vi "AudioTest.Calibrate Generated Waveform, Scale Amplitude based on Frequency.vi"(8 "error in (no error)":errorcluster, 10 "Calibration File":path=path "C:/MTE/Utah Core Audio Test/Config/Speaker Calibration, PN XXX, SN YYY, v10-30-18.csv", 11 "Frequencies and Amplitudes":T1(array[cluster])=[{"frequency [Hz]"=100.0, "amplitude [V]"=1.0}, {"frequency [Hz]"=104.55297296988265, "amplitude [V]"=1.0}, {"frequency [Hz]"=109.31324156841022, "amplitude [V]"=1.0}, {"frequency [Hz]"=114.29024390952246, "amplitude [V]"=1.0}, {"frequency [Hz]"=119.49384782193596, "amplitude [V]"=1.0}, {"frequency [Hz]"=124.93437041394141, "amplitude [V]"=1.0}, {"frequency [Hz]"=130.62259852898134, "amplitude [V]"=1.0}, {"frequency [Hz]"=136.56981013256419, "amplitude [V]"=1.0}, {"frequency [Hz]"=142.78779667291988, "amplitude [V]"=1.0}, {"frequency [Hz]"=149.28888645972907, "amplitude [V]"=1.0}, {"frequency [Hz]"=156.08596910727934, "amplitude [V]"=1.0}, {"frequency [Hz]"=163.19252109051314, "amplitude [V]"=1.0}, {"frequency [Hz]"=170.62263246463442, "amplitude [V]"=1.0}, {"frequency [Hz]"=178.39103480125144, "amplitude [V]"=1.0}, {"frequency [Hz]"=186.51313039644634, "amplitude [V]"=1.0}, {"frequency [Hz]"=195.00502280867852, "amplitude [V]"=1.0}, {"frequency [Hz]"=203.88354878707136, "amplitude [V]"=1.0}, {"frequency [Hz]"=213.1663116533842, "amplitude [V]"=1.0}, {"frequency [Hz]"=222.87171620385857, "amplitude [V]"=1.0}, {"frequency [Hz]"=233.01900520013405, "amplitude [V]"=1.0}, {"frequency [Hz]"=243.6282975215856, "amplitude [V]"=1.0}, {"frequency [Hz]"=254.72062805472865, "amplitude [V]"=1.0}, {"frequency [Hz]"=266.31798939877575, "amplitude [V]"=1.0}, {"frequency [Hz]"=278.4433754700372, "amplitude [V]"=1.0}, {"frequency [Hz]"=291.1208270916169, "amplitude [V]"=1.0}, {"frequency [Hz]"=304.37547965879696, "amplitude [V]"=1.0}, {"frequency [Hz]"=318.233612974613, "amplitude [V]"=1.0}, {"frequency [Hz]"=332.72270335442806, "amplitude [V]"=1.0}, {"frequency [Hz]"=347.871478102818, "amplitude [V]"=1.0}, {"frequency [Hz]"=363.70997247077054, "amplitude [V]"=1.0}, {"frequency [Hz]"=380.2695892061327, "amplitude [V]"=1.0}, {"frequency [Hz]"=397.5831608153717, "amplitude [V]"=1.0}, {"frequency [Hz]"=415.6850146601006, "amplitude [V]"=1.0}, {"frequency [Hz]"=434.61104101742814, "amplitude [V]"=1.0}, {"frequency [Hz]"=454.3987642390772, "amplitude [V]"=1.0}, {"frequency [Hz]"=475.08741715036314, "amplitude [V]"=1.0}, {"frequency [Hz]"=496.7180188365328, "amplitude [V]"=1.0}, {"frequency [Hz]"=519.3334559706973, "amplitude [V]"=1.0}, {"frequency [Hz]"=542.9785678446004, "amplitude [V]"=1.0}, {"frequency [Hz]"=567.700235270821, "amplitude [V]"=1.0}, {"frequency [Hz]"=593.5474735326624, "amplitude [V]"=1.0}, {"frequency [Hz]"=620.5715295660258, "amplitude [V]"=1.0}, {"frequency [Hz]"=648.8259835659542, "amplitude [V]"=1.0}, {"frequency [Hz]"=678.3668552192873, "amplitude [V]"=1.0}, {"frequency [Hz]"=709.2527147740651, "amplitude [V]"=1.0}, {"frequency [Hz]"=741.5447991658872, "amplitude [V]"=1.0}, {"frequency [Hz]"=775.3071334314806, "amplitude [V]"=1.0}, {"frequency [Hz]"=810.6066576501887, "amplitude [V]"=1.0}, {"frequency [Hz]"=847.5133596650709, "amplitude [V]"=1.0}, {"frequency [Hz]"=886.1004138467658, "amplitude [V]"=1.0}, {"frequency [Hz]"=926.4443261752274, "amplitude [V]"=1.0}, {"frequency [Hz]"=968.6250859269978, "amplitude [V]"=1.0}, {"frequency [Hz]"=1012.7263242687566, "amplitude [V]"=1.0}, {"frequency [Hz]"=1058.8354800716002, "amplitude [V]"=1.0}, {"frequency [Hz]"=1107.0439732747873, "amplitude [V]"=1.0}, {"frequency [Hz]"=1157.4473861427032, "amplitude [V]"=1.0}, {"frequency [Hz]"=1210.1456527743937, "amplitude [V]"=1.0}, {"frequency [Hz]"=1265.2432572414218, "amplitude [V]"=1.0}, {"frequency [Hz]"=1322.8494407468877, "amplitude [V]"=1.0}, {"frequency [Hz]"=1383.0784182163372, "amplitude [V]"=1.0}, {"frequency [Hz]"=1446.0496047500092, "amplitude [V]"=1.0}, {"frequency [Hz]"=1511.8878523853718, "amplitude [V]"=1.0}, {"frequency [Hz]"=1580.723697639417, "amplitude [V]"=1.0}, {"frequency [Hz]"=1652.693620321469, "amplitude [V]"=1.0}, {"frequency [Hz]"=1727.9403141296805, "amplitude [V]"=1.0}, {"frequency [Hz]"=1806.612969567712, "amplitude [V]"=1.0}, {"frequency [Hz]"=1888.867569742524, "amplitude [V]"=1.0}, {"frequency [Hz]"=1974.8671996297824, "amplitude [V]"=1.0}, {"frequency [Hz]"=2064.7823694200047, "amplitude [V]"=1.0}, {"frequency [Hz]"=2158.7913525866, "amplitude [V]"=1.0}, {"frequency [Hz]"=2257.080539346032, "amplitude [V]"=1.0}, {"frequency [Hz]"=2359.8448062109383, "amplitude [V]"=1.0}, {"frequency [Hz]"=2467.2879023689043, "amplitude [V]"=1.0}, {"frequency [Hz]"=2579.6228536529447, "amplitude [V]"=1.0}, {"frequency [Hz]"=2697.0723849046813, "amplitude [V]"=1.0}, {"frequency [Hz]"=2819.8693615675606, "amplitude [V]"=1.0}, {"frequency [Hz]"=2948.257251385734, "amplitude [V]"=1.0}, {"frequency [Hz]"=3082.4906071239316, "amplitude [V]"=1.0}, {"frequency [Hz]"=3222.8355712654557, "amplitude [V]"=1.0}, {"frequency [Hz]"=3369.5704036889383, "amplitude [V]"=1.0}, {"frequency [Hz]"=3522.9860333700613, "amplitude [V]"=1.0}, {"frequency [Hz]"=3683.3866352021446, "amplitude [V]"=1.0}, {"frequency [Hz]"=3851.090233079168, "amplitude [V]"=1.0}, {"frequency [Hz]"=4026.429330437053, "amplitude [V]"=1.0}, {"frequency [Hz]"=4209.751569503279, "amplitude [V]"=1.0}, {"frequency [Hz]"=4401.4204205619735, "amplitude [V]"=1.0}, {"frequency [Hz]"=4601.81590260106, "amplitude [V]"=1.0}, {"frequency [Hz]"=4811.3353367702475, "amplitude [V]"=1.0}, {"frequency [Hz]"=5030.394134143814, "amplitude [V]"=1.0}, {"frequency [Hz]"=5259.426619349943, "amplitude [V]"=1.0}, {"frequency [Hz]"=5498.886891699759, "amplitude [V]"=1.0}, {"frequency [Hz]"=5749.249725523269, "amplitude [V]"=1.0}, {"frequency [Hz]"=6011.011511497396, "amplitude [V]"=1.0}, {"frequency [Hz]"=6284.691240832413, "amplitude [V]"=1.0}, {"frequency [Hz]"=6570.831534268094, "amplitude [V]"=1.0}, {"frequency [Hz]"=6869.9997179198535, "amplitude [V]"=1.0}, {"frequency [Hz]"=7182.788948107758, "amplitude [V]"=1.0}, {"frequency [Hz]"=7509.819387398822, "amplitude [V]"=1.0}, {"frequency [Hz]"=7851.739434194097, "amplitude [V]"=1.0}, {"frequency [Hz]"=8209.22700829857, "amplitude [V]"=1.0}, {"frequency [Hz]"=8582.99089502272, "amplitude [V]"=1.0}, {"frequency [Hz]"=8973.772150480592, "amplitude [V]"=1.0}, {"frequency [Hz]"=9382.345570870839, "amplitude [V]"=1.0}, {"frequency [Hz]"=9809.52122865357, "amplitude [V]"=1.0}, {"frequency [Hz]"=10256.146078669068, "amplitude [V]"=1.0}, {"frequency [Hz]"=10723.105637382549, "amplitude [V]"=1.0}, {"frequency [Hz]"=11211.32573858456, "amplitude [V]"=1.0}, {"frequency [Hz]"=11721.774369027788, "amplitude [V]"=1.0}, {"frequency [Hz]"=12255.46358764028, "amplitude [V]"=1.0}, {"frequency [Hz]"=12813.451532119352, "amplitude [V]"=1.0}, {"frequency [Hz]"=13396.84451688576, "amplitude [V]"=1.0}, {"frequency [Hz]"=14006.799226556774, "amplitude [V]"=1.0}, {"frequency [Hz]"=14644.525009287636, "amplitude [V]"=1.0}, {"frequency [Hz]"=15311.286274528236, "amplitude [V]"=1.0}, {"frequency [Hz]"=16008.404999948825, "amplitude [V]"=1.0}, {"frequency [Hz]"=16737.26335250587, "amplitude [V]"=1.0}, {"frequency [Hz]"=17499.306428843538, "amplitude [V]"=1.0}, {"frequency [Hz]"=18296.04512046572, "amplitude [V]"=1.0}, {"frequency [Hz]"=19129.059109358055, "amplitude [V]"=1.0}, {"frequency [Hz]"=20000.0, "amplitude [V]"=1.0}]) -> (0 "error out":errorcluster, 3 "Frequencies and Amplitudes Out":T1(array[cluster]))   [LabVIEW 2018]
uses:
  <vilib>/KATE/Files/File Utils.lvlib
panel:
  in  "Normal":bool=TRUE
  out "Cnt":i32
  out "XY Graph":cluster{dbl[], dbl[]}[](graph)
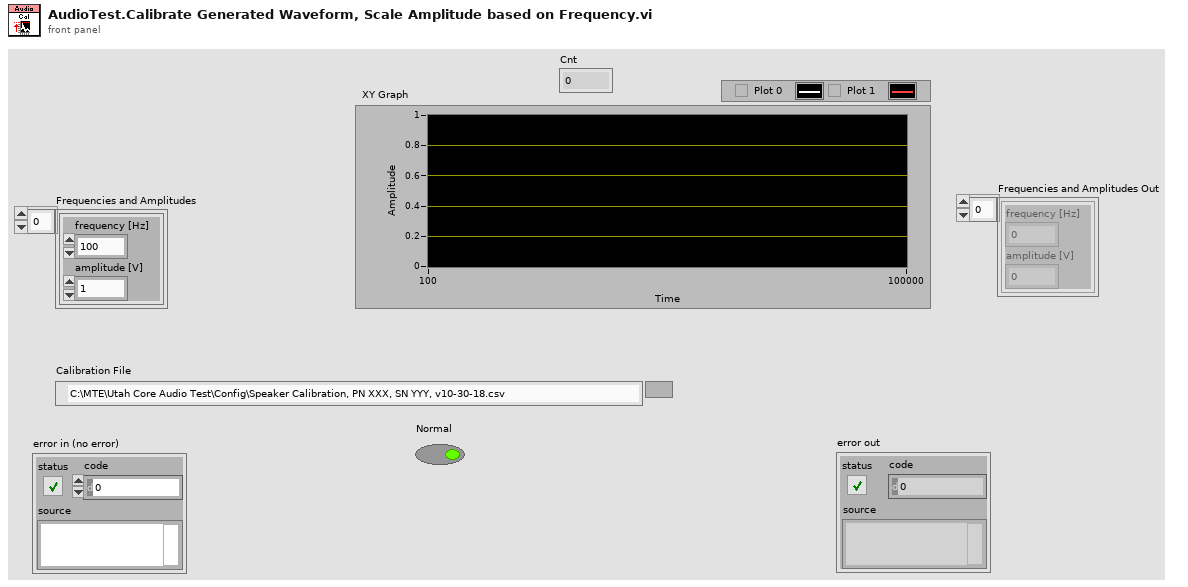
[diagram p1: front panel]
types:
  T1 = cluster{"frequency [Hz]":dbl, "amplitude [V]":dbl}[]
  T2 = cluster{"frequency [Hz]":dbl, "amplitude [V]":dbl}
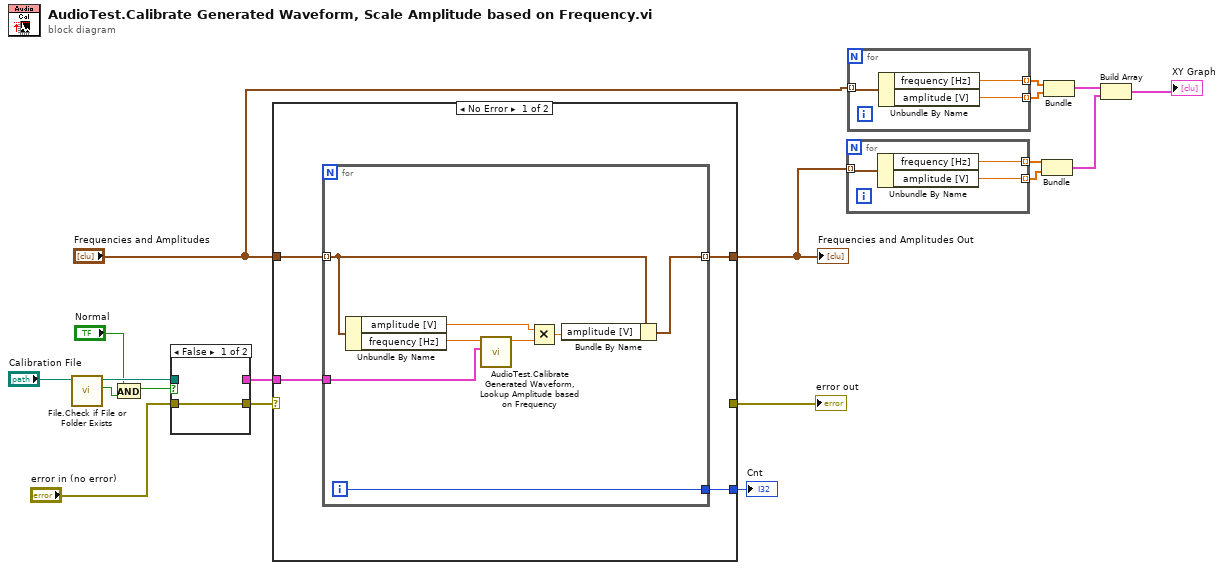
[diagram p0: block diagram]
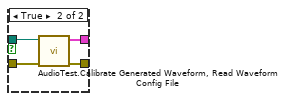
[diagram p2: hidden frame]
diagram:
  n1 = call <vilib>:"File.Check if File or Folder Exists.vi"("Path"="Calibration File") -> ("Exists"=w2:bool, "Dup Path"=w5:path)  [unwired: 6 in, 3 out]
  n2 = And(x="Normal", y=w2) -> (x .and. y?=w3:bool)
  n3 = case shown="False" w3 {
    tunnel: w5 -> [_ w24]
    tunnel: "error in (no error)" -> [w20 w23]
    tunnel: [w20 w22] -> w18
    tunnel: [_ w21] -> w17
    frame False {
    }
    frame True {
      n4 = call "AudioTest.Calibrate Generated Waveform, Read Waveform Config File.vi"("error in"=w23, "Config File"=w24) -> ("error out"=w22:errorcluster, "Waveform Cal"=w21:cluster{"Freq":dbl[], "Gain":dbl[]})  [unwired: 8 in]
    }
  }
  n5 = case shown="No Error" w18 {
    selector: w18 -> [_ w38]
    tunnel: "Frequencies and Amplitudes" -> [w28 w37]
    tunnel: [w27 w37] -> w10
    tunnel: w17 -> [w26 _]
    tunnel: [_ w38] -> w16
    tunnel: [w25 _] -> w4
    frame No Error {
      n6 = for {
        tunnel: w28 -> [w30] mode=indexing
        tunnel: [w31] -> w27 mode=indexing
        tunnel: w26 -> [w35]
        tunnel: [w29] -> w25
        i -> [w29]
        n7 = Unbundle By Name(w30) -> ("amplitude [V]"=w33:dbl, "frequency [Hz]"=w36:dbl)
        n8 = call "AudioTest.Calibrate Generated Waveform, Lookup Amplitude based on Frequency.vi"("Waveform Cal"=w35, "Freq"=w36) -> ("Gain"=w34:dbl)  [unwired: 9 in]
        n9 = Multiply(x=w33, y=w34) -> (x*y=w32:dbl)
        n10 = Bundle By Name(cluster=w30, "amplitude [V]"=w32) -> (w31:T2)
      }
    }
    frame Error {
    }
  }
  "Frequencies and Amplitudes Out" <- w10
  "error out" <- w16
  "Cnt" <- w4
  n11 = for {
    tunnel: w10 -> [w41] mode=indexing
    tunnel: [w40] -> w9 mode=indexing
    tunnel: [w39] -> w8 mode=indexing
    n12 = Unbundle By Name(w41) -> ("frequency [Hz]"=w40:dbl, "amplitude [V]"=w39:dbl)
  }
  n13 = for {
    tunnel: "Frequencies and Amplitudes" -> [w44] mode=indexing
    tunnel: [w43] -> w14 mode=indexing
    tunnel: [w42] -> w13 mode=indexing
    n14 = Unbundle By Name(w44) -> ("frequency [Hz]"=w43:dbl, "amplitude [V]"=w42:dbl)
  }
  n15 = Bundle(w9, w8) -> (w7:cluster{dbl[], dbl[]})  [unwired: 1 in]
  n16 = Bundle(w14, w13) -> (w12:cluster{dbl[], dbl[]})  [unwired: 1 in]
  n17 = Build Array(w12, w7) -> (→"XY Graph":cluster{dbl[], dbl[]}[])
